vi "Begin.vi"(8 "error in":errorcluster) -> (0 "error out":errorcluster)   [LabVIEW 2016]
doc: "Called before other user functions, this VI is expected to open initial I/O refnums, load in file data, and do all program initialization. Notice that the <B>error out</B> terminal is simply used for data flow. Wiring it to other structures or subVIs ensures that this VI runs first."
uses:
  <vilib>/Rock Robotics/SystemInterfaces/DIO/FPGA_DIOPWMChannel.ctl
  <vilib>/Rock Robotics/WPI/SafetyOutput/WPI_SafetyOutputConfigMenu.ctl
  <vilib>/Rock Robotics/WPI/DriverStation/WPI_DriverStationRobotMode2.ctl
  <vilib>/Rock Robotics/WPI/Joystick/WPI_JoystickDeviceEnum.ctl
  <vilib>/Rock Robotics/WPI/Accelerometer/WPI_AccelerometerRange.ctl
  <vilib>/Rock Robotics/SystemInterfaces/spilib/spi_bus.ctl
  <vilib>/Rock Robotics/WPI/Relay/WPI_RelayDirection.ctl
  <vilib>/Rock Robotics/SystemInterfaces/DIO/FPGA_DIORelayChannel.ctl
  <vilib>/Rock Robotics/WPI/RobotDrive/WPI_RobotDriveOpen2MotorWithSPARK.vi
  Robot Global Data.vi
  <vilib>/Rock Robotics/Network Tables/NT Write String Array.vi
  <vilib>/Rock Robotics/WPI/Accelerometer/InternalAccelerometer/WPI_AccelerometerInternalOpen.vi
  <vilib>/Rock Robotics/WPI/Gyro/WPI_GyroXRS450_SPI_Open.vi
  <vilib>/Rock Robotics/WPI/MotorControl/WPI_MotorControlOpen SPARK.vi
  <vilib>/Rock Robotics/SystemInterfaces/DIO/FPGA_DIOChannel.ctl
  <vilib>/Rock Robotics/WPI/Counter/WPI_CounterDigitalInputToDigitalSource.vi
  <vilib>/Rock Robotics/WPI/Encoder/WPI_EncoderType.ctl
  <vilib>/Rock Robotics/WPI/Switch/WPI_SwitchOpenLimit.vi
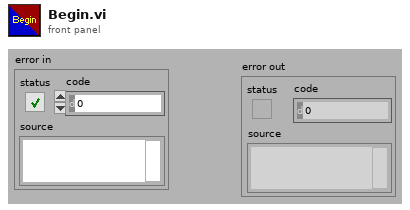
[diagram p1: front panel]
types:
  T1 = typedef "FPGA_DIOPWMChannel.ctl" = enum8{"PWM 0", "PWM 1", "PWM 2", "PWM 3", "PWM 4", "PWM 5", "PWM 6", "PWM 7", "PWM 8", "PWM 9", "PWM MXP 0", "PWM MXP 1", "PWM MXP 2", "PWM MXP 3", "PWM MXP 4", "PWM MXP 5", "PWM MXP 6", "PWM MXP 7", "PWM MXP 8", "PWM MXP 9", "Invalid"}
  T2 = typedef "FPGA_DIORelayChannel.ctl" = enum8{"Relay 0", "Relay 1", "Relay 2", "Relay 3", "Invalid"}
  T3 = typedef "WPI_RelayDirection.ctl" = enum16{"Both directions", "Forward only", "Reverse only"}
  T4 = typedef "spi_bus.ctl" = enum16{"SPI On-Board, CS0", "SPI On-Board, CS1", "SPI On-Board, CS2", "SPI On-Board, CS3", "SPI MXP", "Invalid"}
  T5 = typedef "WPI_AccelerometerRange.ctl" = enum16{"+/- 2 g", "+/- 4 g", "+/- 8 g"}
  T6 = typedef "WPI_JoystickDeviceEnum.ctl" = enum16{"USB 0", "USB 1", "USB 2", "USB 3", "USB 4", "USB 5"}
  T7 = typedef "WPI_DriverStationRobotMode2.ctl" = enum16{"Autonomous Disabled", "Autonomous Enabled", "Teleop Disabled", "Teleop Enabled", "Disconnected", "Finish", "Test Disabled", "Test Enabled", "Emergency Stopped"}
  T8 = typedef "WPI_SafetyOutputConfigMenu.ctl" = enum16{"Enable", "Disable"}
  T9 = typedef "WPI_ServoDeviceRef.ctl" = cluster{"DeviceStatus":errorcluster, "PWM Channel":T1, "DeadBand":T10}
  T10 = typedef "WPI_PWMDeadband.ctl" = cluster{"Name":string, "maxPositivePwm":i32, "minPositivePwm":i32, "centerPwm":i32, "maxNegativePwm":i32, "minNegativePwm":i32, "angularRange":u16}
  T11 = typedef "FPGA_DIOChannel.ctl" = enum8{"DIO 0", "DIO 1", "DIO 2", "DIO 3", "DIO 4", "DIO 5", "DIO 6", "DIO 7", "DIO 8", "DIO 9", "DIO MXP 0", "DIO MXP 1", "DIO MXP 2", "DIO MXP 3", "DIO MXP 4", "DIO MXP 5", "DIO MXP 6", "DIO MXP 7", "DIO MXP 8", "DIO MXP 9", "DIO MXP 10", "DIO MXP 11", "DIO MXP 12", "DIO MXP 13", "DIO MXP 14", "DIO MXP 15", "SPI Port CS1", "SPI Port CS2", "SPI Port CS3", "SPI Port MISO", "SPI Port MOSI", "Invalid"}
  T12 = typedef "WPI_SwitchDevRef.ctl" = cluster{"DevStatus":errorcluster, "DIO Channel":T11, "CntIndex":T13, "Normally Closed":bool}
  T13 = typedef "FPGA_CounterCtrSystemIndex.ctl" = enum8{"Ctr 0", "Ctr 1", "Ctr 2", "Ctr 3", "Ctr 4", "Ctr 5", "Ctr 6", "Ctr 7", "Invalid"}
  T14 = typedef "WPI_EncoderType.ctl" = enum16{"1x", "2x", "4x"}
  T15 = typedef "WPI_DigitalInputDevRef.ctl" = cluster{"DevStatus":errorcluster, "DIO Channel":T11}
  T16 = typedef "FPGA_CounterEncoderSourceConvertionLVSourceType.ctl" = cluster{"DevStatus":errorcluster, "AnalogTriggerMode?":bool, "DigitalMode":cluster{"DIO Channel":T17}, "AnalogTriggerMode":cluster{"AnalogTriggerIndex":T18, "OutputType":T19}}
  T17 = typedef "FPGA_DIODigitalSourceChannel.ctl" = enum8{"DIO 0", "DIO 1", "DIO 2", "DIO 3", "DIO 4", "DIO 5", "DIO 6", "DIO 7", "DIO 8", "DIO 9", "DIO MXP 0", "DIO MXP 1", "DIO MXP 2", "DIO MXP 3", "DIO MXP 4", "DIO MXP 5", "DIO MXP 6", "DIO MXP 7", "DIO MXP 8", "DIO MXP 9", "DIO MXP 10", "DIO MXP 11", "DIO MXP 12", "DIO MXP 13", "DIO MXP 14", "DIO MXP 15", "Disabled"}
  T18 = typedef "FPGA_AnalogTriggerIndex.ctl" = enum8{"Trig 0", "Trig 1", "Trig 2", "Trig 3", "Trig 4", "Trig 5", "Trig 6", "Trig 7", "Invalid"}
  T19 = typedef "FPGA_AnalogTriggerOutType.ctl" = enum16{"InWindow", "TriggerState", "Rising", "Falling"}
  T20 = typedef "WPI_EncoderDevRef.ctl" = cluster{"DevStatus":errorcluster, "EncoderIndex":T21, "CounterIndex":T13, "DistancePerCount":dbl, "Decoding Type":T14}
  T21 = typedef "FPGA_EncoderIdx.ctl" = enum8{"Enc 0", "Enc 1", "Enc 2", "Enc 3", "Enc 4", "Enc 5", "Enc 6", "Enc 7", "Invalid"}
  T22 = typedef "WPI_JoystickDevRef.ctl" = cluster{"Device":T6}
  T23 = typedef "WPI_RobotDriveDevRef.ctl" = cluster{"DevStatus":errorcluster, "Motors[]":T24[], "Square Inputs":bool, "Max Output":dbl}
  T24 = typedef "WPI_MotorControlDeviceRef.ctl" = cluster{"DeviceStatus":errorcluster, "Type":T25, "PWM":cluster{"PWM Channel":T1, "DeadBand":T10}, "CAN":cluster{"Device Number":u8, "SetOutput VI Ref":variant, "GetOutput VI Ref":variant, "Enable VI Ref":variant, "Disable VI Ref":variant, "Data":variant}, "Invert":bool}
  T25 = typedef "WPI_MotorControlType.ctl" = enum16{"PWM", "CAN"}
  T26 = typedef "WPI_RelayDevRef.ctl" = cluster{"DevStatus":errorcluster, "Relay Channel":T2, "Relay Direction":T3}
  T27 = typedef "WPI_GyroDevRef.ctl" = cluster{"DevStatus":errorcluster, "Analog Channel":T28, "Offset":dbl, "Gain (VoltsPerDegree/Second)":dbl, "Gyro Type":enum16{"Analog", "XRS450"}, "Handle":i32, "SPI Bus":T4, "Device Found":bool, "Sample Rate":dbl, "Calibrate On Open":bool}
  T28 = typedef "FPGA_AIChannel.ctl" = enum8{"AI 0", "AI 1", "AI 2", "AI 3", "AI MXP 0", "AI MXP 1", "AI MXP 2", "AI MXP 3", "Invalid"}
  T29 = typedef "WPI_AccelerometerDevRef.ctl" = cluster{"DevStatus":errorcluster, "Scaling":T30, "Analog Channels":T31, "I2C Bus":T32, "SPI Bus":T4, "Accel Range":T33, "ADXL Axes":T34, "Handle":i32, "Device Address":u8, "Accel Type":enum16{"Analog", "ADXL345 I2C", "ADXL345 SPI", "Internal", "ADXL362 SPI"}}
  T30 = typedef "WPI_AccelerometerScaling.ctl" = cluster{"Gain (VoltsPerG)":dbl, "Center Voltage":dbl}
  T31 = typedef "WPI_AccelerometerAnalogChannels.ctl" = cluster{"X-Axis":T28, "Y-Axis":T28, "Z-Axis":T28}
  T32 = typedef "i2c_bus.ctl" = enum16{"I2C On-Board", "I2C MXP", "Invalid"}
  T33 = typedef "ADXL345 Range.ctl" = u8
  T34 = typedef "WPI_AccelerometerADXL345 Axes.ctl" = cluster{"X-Axis":bool, "Y-Axis":bool, "Z-Axis":bool}
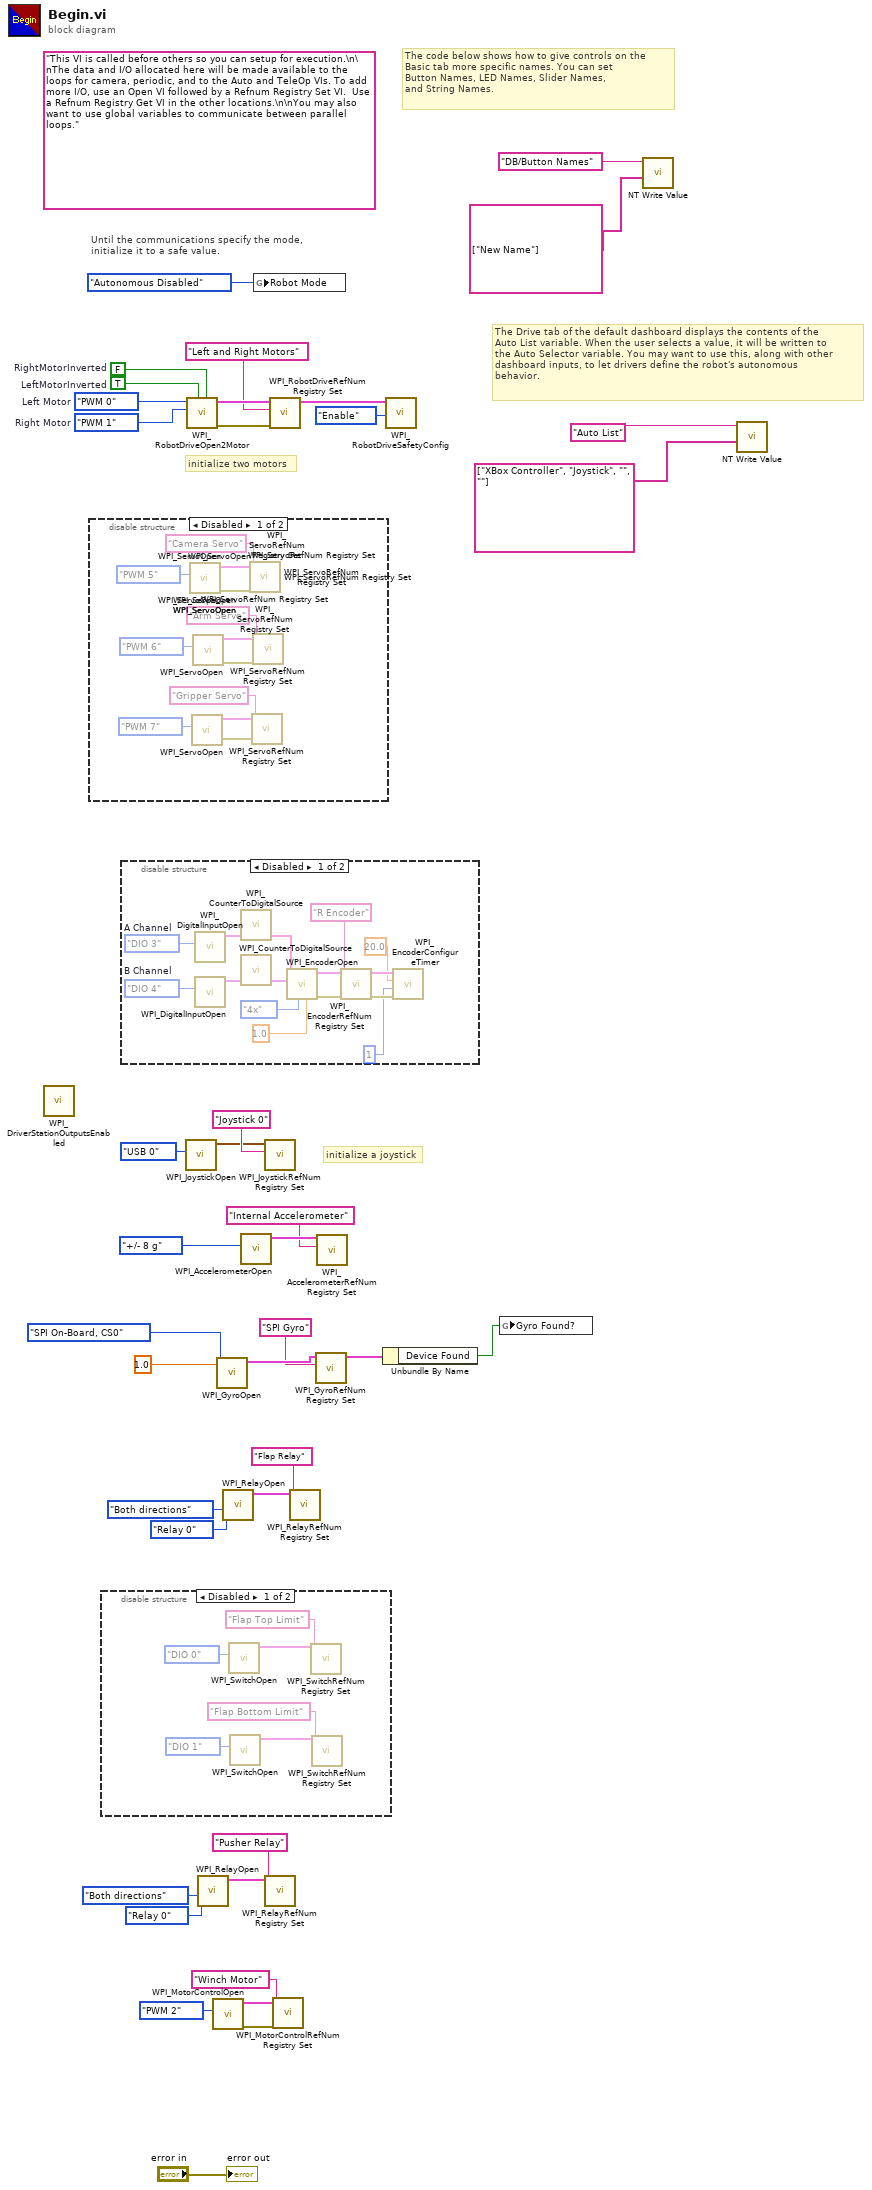
[diagram p0: block diagram]
diagram:
  (unwired) "This VI is called before others so you can setup for execution.\n\nThe data and I/O allocated here will be made available to the loops for camera, periodic, and to the Auto and TeleOp VIs. To add more I/O, use an Open VI followed by a Refnum Registry Set VI.  Use a Refnum Registry Get VI in the other locations.\n\nYou may also want to use global variables to communicate between parallel loops."
  w33 = FPGA_DIOPWMChannel."PWM 1"  # Right Motor
  w34 = FPGA_DIOPWMChannel."PWM 0"  # Left Motor
  w38 = TRUE  # LeftMotorInverted
  w39 = FALSE  # RightMotorInverted
  # "The Drive tab of the default dashboard displays the contents of the\nAuto List variable. When the user selects a value, it will be written to\nthe Auto Selector variable. You may want to use this, along with other\ndashboard inputs, to let drivers define the robot's autonomous\nbehavior."
  # "The code below shows how to give controls on the\nBasic tab more specific names. You can set\nButton Names, LED Names, Slider Names,\nand String Names."
  # "initialize a joystick"
  # "Until the communications specify the mode,\ninitialize it to a safe value."
  # "initialize two motors"
  n1 = call <vilib>:"WPI_DriverStationOutputsEnabled.vi"() -> ()  [unwired: 10 in, 2 out]
  n2 = disable-structure shown="Disabled" {
    frame Disabled {
      n3 = call <vilib>:"WPI_ServoOpen.vi"("PWM Channel"=FPGA_DIOPWMChannel."PWM 5") -> ("error out"=w41:errorcluster, "ServoDeviceRef"=w42:T9)  [unwired: 9 in]
      n4 = call <vilib>:"WPI_ServoOpen.vi"("PWM Channel"=FPGA_DIOPWMChannel."PWM 5") -> ("error out"=w46:errorcluster, "ServoDeviceRef"=w45:T9)  [unwired: 9 in]
      n5 = call <vilib>:"WPI_ServoOpen.vi"("PWM Channel"=FPGA_DIOPWMChannel."PWM 5") -> ("error out"=w49:errorcluster, "ServoDeviceRef"=w50:T9)  [unwired: 9 in]
      n6 = call <vilib>:"WPI_ServoOpen.vi"("PWM Channel"=FPGA_DIOPWMChannel."PWM 5") -> ("error out"=w54:errorcluster, "ServoDeviceRef"=w53:T9)  [unwired: 9 in]
      n7 = call <vilib>:"WPI_ServoOpen.vi"("PWM Channel"=FPGA_DIOPWMChannel."PWM 5") -> ("error out"=w57:errorcluster, "ServoDeviceRef"=w58:T9)  [unwired: 9 in]
      n8 = call <vilib>:"WPI_ServoOpen.vi"("PWM Channel"=FPGA_DIOPWMChannel."PWM 5") -> ("error out"=w70:errorcluster, "ServoDeviceRef"=w69:T9)  [unwired: 9 in]
      n9 = call <vilib>:"WPI_ServoOpen.vi"("PWM Channel"=FPGA_DIOPWMChannel."PWM 7") -> ("error out"=w62:errorcluster, "ServoDeviceRef"=w61:T9)  [unwired: 9 in]
      n10 = call <vilib>:"WPI_ServoOpen.vi"("PWM Channel"=FPGA_DIOPWMChannel."PWM 6") -> ("error out"=w65:errorcluster, "ServoDeviceRef"=w66:T9)  [unwired: 9 in]
      n11 = call <vilib>:"WPI_ServoRefNum Registry Set.vi"("error in (no error)"=w41, "refnum name"="Camera Servo", "ServoDeviceRef"=w42) -> ()  [unwired: 7 in, 2 out]
      n12 = call <vilib>:"WPI_ServoRefNum Registry Set.vi"("error in (no error)"=w46, "refnum name"="Camera Servo", "ServoDeviceRef"=w45) -> ()  [unwired: 7 in, 2 out]
      n13 = call <vilib>:"WPI_ServoRefNum Registry Set.vi"("error in (no error)"=w49, "refnum name"="Camera Servo", "ServoDeviceRef"=w50) -> ()  [unwired: 7 in, 2 out]
      n14 = call <vilib>:"WPI_ServoRefNum Registry Set.vi"("error in (no error)"=w54, "refnum name"="Camera Servo", "ServoDeviceRef"=w53) -> ()  [unwired: 7 in, 2 out]
      n15 = call <vilib>:"WPI_ServoRefNum Registry Set.vi"("error in (no error)"=w57, "refnum name"="Camera Servo", "ServoDeviceRef"=w58) -> ()  [unwired: 7 in, 2 out]
      n16 = call <vilib>:"WPI_ServoRefNum Registry Set.vi"("error in (no error)"=w70, "refnum name"="Camera Servo", "ServoDeviceRef"=w69) -> ()  [unwired: 7 in, 2 out]
      n17 = call <vilib>:"WPI_ServoRefNum Registry Set.vi"("error in (no error)"=w62, "refnum name"="Gripper Servo", "ServoDeviceRef"=w61) -> ()  [unwired: 7 in, 2 out]
      n18 = call <vilib>:"WPI_ServoRefNum Registry Set.vi"("error in (no error)"=w65, "refnum name"="Arm Servo", "ServoDeviceRef"=w66) -> ()  [unwired: 7 in, 2 out]
    }
    frame Enabled {
    }
  }
  n19 = disable-structure shown="Disabled" {
    frame Disabled {
      n20 = call-poly <vilib>:"WPI_SwitchOpen.vi"("DIO Channel"=FPGA_DIOChannel."DIO 0") -> ("SwitchDevRef"=w76:T12)  [unwired: 9 in, 1 out]
      n21 = call-poly <vilib>:"WPI_SwitchOpen.vi"("DIO Channel"=FPGA_DIOChannel."DIO 1") -> ("SwitchDevRef"=w73:T12)  [unwired: 9 in, 1 out]
      n22 = call <vilib>:"WPI_SwitchRefNum Registry Set.vi"("refnum name"="Flap Top Limit", "SwitchDevRef"=w76) -> ()  [unwired: 8 in, 2 out]
      n23 = call <vilib>:"WPI_SwitchRefNum Registry Set.vi"("refnum name"="Flap Bottom Limit", "SwitchDevRef"=w73) -> ()  [unwired: 8 in, 2 out]
    }
    frame Enabled {
    }
  }
  n24 = disable-structure shown="Disabled" {
    frame Disabled {
      w92 = FPGA_DIOChannel."DIO 4"  # B Channel
      w91 = FPGA_DIOChannel."DIO 3"  # A Channel
      n25 = call <vilib>:"WPI_DigitalInputOpen.vi"("DIO Channel"=w91) -> ("DigitalInputDevRef"=w88:T15)  [unwired: 1 in, 9 out]
      n26 = call <vilib>:"WPI_DigitalInputOpen.vi"("DIO Channel"=w92) -> ("DigitalInputDevRef"=w89:T15)  [unwired: 1 in, 9 out]
      n27 = call-poly <vilib>:"WPI_CounterToDigitalSource.vi"("DigitalInputDevRef"=w88) -> ("Digital Source"=w87:T16)  [unwired: 6 out]
      n28 = call-poly <vilib>:"WPI_CounterToDigitalSource.vi"("DigitalInputDevRef"=w89) -> ("Digital Source"=w90:T16)  [unwired: 6 out]
      n29 = call <vilib>:"WPI_EncoderOpen.vi"("DistancePerCount"=1.0, "Decoding Type"=WPI_EncoderType."4x", "BSource"=w90, "ASource"=w87) -> ("error out"=w84:errorcluster, "EncoderDevRef"=w83:T20)  [unwired: 4 in, 2 out]
      n30 = call <vilib>:"WPI_EncoderRefNum Registry Set.vi"("error in (no error)"=w84, "refnum name"="R Encoder", "EncoderDevRef"=w83) -> ("error out"=w81:errorcluster, "EncoderDevRef"=w80:T20)  [unwired: 7 in]
      n31 = call <vilib>:"WPI_EncoderConfigureTimer.vi"("error in (no error)"=w81, "Number Samples to Average"=u8 1, "Minimum Rate"=20.0, "EncoderDevRef"=w80) -> ()  [unwired: 6 in, 2 out]
    }
    frame Enabled {
    }
  }
  n32 = call <vilib>:"WPI_JoystickOpen.vi"("JoystickDevice"=WPI_JoystickDeviceEnum."USB 0") -> ("JoystickDevRef"=w28:T22)  [unwired: 10 in]
  n33 = call-poly <vilib>:"WPI_RobotDriveOpen2Motor.vi"("Right Motor Inverted"=w39, "Left Motor Inverted"=w38, "Right Motor"=w33, "Left Motor"=w34) -> ("error out"=w35:errorcluster, "RobotDriveDevRef"=w37:T23)  [unwired: 1 in, 5 out]
  n34 = call <vilib>:"WPI_RelayOpen.vi"("Relay Direction"=WPI_RelayDirection."Both directions", "Relay Channel"=FPGA_DIORelayChannel."Relay 0") -> ("RelayDevRef"=w8:T26)  [unwired: 8 in, 1 out]
  n35 = call-poly <vilib>:"WPI_MotorControlOpen.vi"("PWM Channel"=FPGA_DIOPWMChannel."PWM 2") -> ("error out"=w4:errorcluster, "MotorControlDeviceRef"=w1:T24)  [unwired: 9 in]
  n36 = call-poly <vilib>:"WPI_GyroOpen.vi"("Sample Rate (ms)"=1.0, "SPI Bus"=spi_bus."SPI On-Board, CS0") -> ("GyroDevRef"=w19:T27)  [unwired: 8 in, 1 out]
  n37 = call <vilib>:"WPI_RelayOpen.vi"("Relay Direction"=WPI_RelayDirection."Both directions", "Relay Channel"=FPGA_DIORelayChannel."Relay 0") -> ("RelayDevRef"=w11:T26)  [unwired: 8 in, 1 out]
  n38 = call-poly <vilib>:"WPI_AccelerometerOpen.vi"("Accel Range"=WPI_AccelerometerRange."+/- 8 g") -> ("AccelerometerDevRef"=w21:T29)  [unwired: 9 in, 1 out]
  n39 = global write "Robot Global Data.vi" "Robot Mode"(WPI_DriverStationRobotMode2."Autonomous Disabled" ("Robot Mode")) -> ()
  n40 = call <vilib>:"WPI_JoystickRefNum Registry Set.vi"("refnum name"="Joystick 0", "JoystickDevRef"=w28) -> ()  [unwired: 8 in, 2 out]
  n41 = call <vilib>:"WPI_RelayRefNum Registry Set.vi"("refnum name"="Pusher Relay", "RelayDevRef"=w8) -> ()  [unwired: 8 in, 2 out]
  n42 = call <vilib>:"WPI_RobotDriveRefNum Registry Set.vi"("error in (no error)"=w35, "refnum name"="Left and Right Motors", "RobotDriveDevRef"=w37) -> ("RobotDriveDevRef"=w32:T23)  [unwired: 1 in, 7 out]
  n43 = call <vilib>:"WPI_MotorControlRefNum Registry Set.vi"("error in (no error)"=w4, "refnum name"="Winch Motor", "MotorControlDevRef"=w1) -> ()  [unwired: 7 in, 2 out]
  n44 = call <vilib>:"WPI_RelayRefNum Registry Set.vi"("refnum name"="Flap Relay", "RelayDevRef"=w11) -> ()  [unwired: 8 in, 2 out]
  n45 = call <vilib>:"WPI_GyroRefNum Registry Set.vi"("refnum name"="SPI Gyro", "GyroDevRef"=w19) -> ("GyroDevRef"=w15:T27)  [unwired: 8 in, 1 out]
  n46 = call <vilib>:"WPI_AccelerometerRefNum Registry Set.vi"("refnum name"="Internal Accelerometer", "AccelerometerDevRef"=w21) -> ()  [unwired: 8 in, 2 out]
  n47 = Unbundle By Name(w15) -> ("Device Found"=w14:bool)
  n48 = call <vilib>:"WPI_RobotDriveSafetyConfig.vi"("mode"=WPI_SafetyOutputConfigMenu."Enable", "RobotDriveDevRef"=w32) -> ()  [unwired: 8 in, 2 out]
  n49 = global write "Robot Global Data.vi" "Gyro Found?"(w14) -> ()
  n50 = call-poly <vilib>:"NT Write Value.vi"("String Array"=string[] ["New Name"], "Name"="DB/Button Names") -> ()  [unwired: 9 in, 1 out]
  n51 = call-poly <vilib>:"NT Write Value.vi"("String Array"=string[] ["XBox Controller", "Joystick", "", ""], "Name"="Auto List") -> ()  [unwired: 9 in, 1 out]
  "error out" <- "error in"
